vi "Cal_Open_Message_Box.vi"(7 "message":string, 10 "timeout, msec (10000)":u32=5000) -> ()   [LabVIEW 2020]
panel:
  out "message 2":string
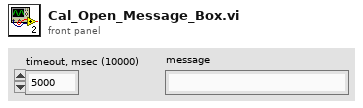
[diagram p1: front panel]
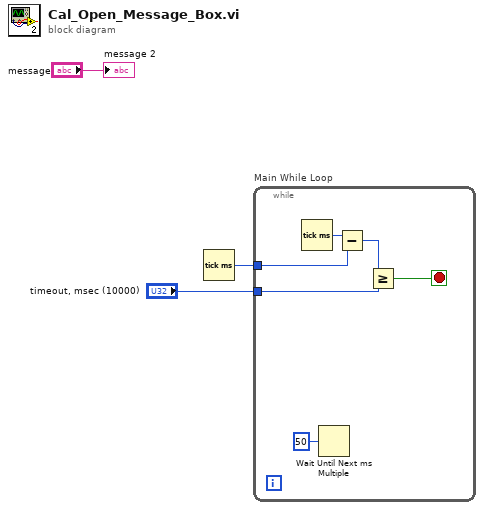
[diagram p0: block diagram]
diagram:
  n1 = Tick Count (ms)() -> (millisecond timer value=w3:u32)
  n2 = while "Main While Loop" {
    tunnel: w3 -> [w7]
    tunnel: "timeout, msec (10000)" -> [w6]
    stop <- w5 stop-if-true
    n3 = Tick Count (ms)() -> (millisecond timer value=w9:u32)
    n4 = Wait Until Next ms Multiple(millisecond multiple=u32 50) -> ()  [unwired: 1 out]
    n5 = Subtract(x=w9, y=w7) -> (x-y=w8:u32)
    n6 = Greater Or Equal?(x=w8, y=w6) -> (x >= y?=w5:bool)
  }
  "message 2" <- "message"
